vi "Lakeshore 370 - Init.vi"(8 "error in (no error)":errorcluster, 11 "Enum":enum16{"Sample stage", "Mixing chamber"}(ring)=enum."Mixing chamber") -> (0 "error out":errorcluster, 3 "VISA resource name out":refnum<visa-resource-name>)   [LabVIEW 2019]
uses:
  _Global variables 1.vi
  <instrlib>/Lake Shore Cryotronics 370/Lake Shore Cryotronics 370.lvlib
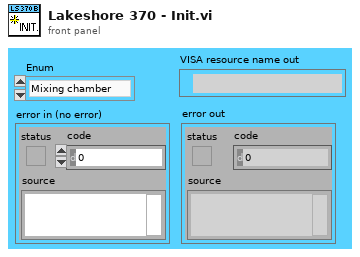
[diagram p1: front panel]
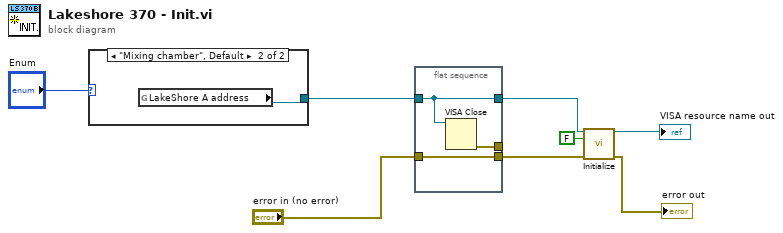
[diagram p0: block diagram]
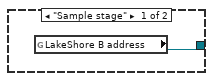
[diagram p2: hidden frame]
diagram:
  n1 = case shown="\"Mixing chamber\", Default" "Enum" {
    tunnel: [w9 w10] -> w5
    frame "Sample stage" {
      n2 = global read "_Global variables 1.vi" "LakeShore B address"() -> (w9:refnum<visa-resource-name>)
    }
    frame "Mixing chamber", Default {
      n3 = global read "_Global variables 1.vi" "LakeShore A address"() -> (w10:refnum<visa-resource-name>)
    }
  }
  n4 = flat-sequence {
    tunnel: w5 -> [w12]
    tunnel: "error in (no error)" -> [w13]
    tunnel: [w13] -> w2
    tunnel: [w12] -> w4
    tunnel: [w11] -> _
    frame #0 {
      n5 = VISA Close(VISA resource name=w12) -> (error out=w11:errorcluster)  [unwired: 1 in]
    }
  }
  n6 = call <instrlib>:"Initialize.vi"("VISA resource name"=w4, "ID Query (True)"=FALSE, "error in (no error)"=w2) -> ("VISA resource name out"=→"VISA resource name out":refnum<visa-resource-name>, "error out"=→"error out":errorcluster)  [unwired: 11 in]
